vi "Generator DC Sweep Manager.vi"(8 "error in (no error)":errorcluster, 10 "sweep index":i32=-1, 11 "Lockin.DAQ in":refnum<class "Lockin.DAQ.lvclass">) -> (0 "error out":errorcluster, 2 "Array":waveform(dbl)[](array[waveform]), 3 "Lockin.DAQ out":refnum<class "Lockin.DAQ.lvclass">)   [LabVIEW 2019, in "Lockin.DAQ.lvclass"]
uses:
  Lockin.DAQ.lvclass
  Lockin.DAQ.lvclass/Lockin.DAQ.ctl
panel:
  out "time":dbl
  out "sweeping":dbl
  out "start sweep time":timestamp
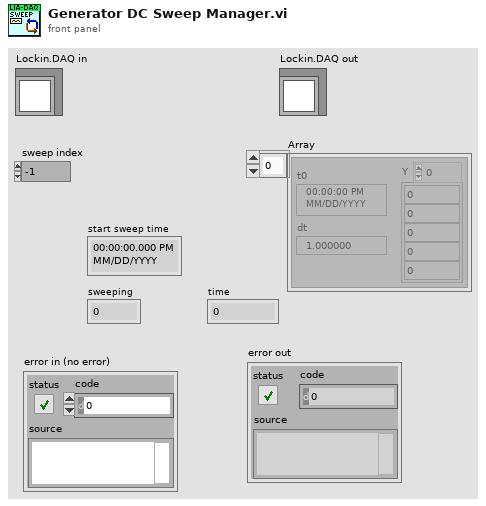
[diagram p1: front panel]
types:
  T1 = typedef "Lockin.DAQ.lvclass/Sampling.ctl" = cluster{"Fs":dbl, "#s":i32}
  T2 = typedef "Lockin.DAQ.lvclass/AO-cluster.ctl" = T3[]
  T3 = typedef "Instrument.Lockin.UI.lvclass/AO Channel--Cluster.ctl" = cluster{"Enable?":bool, "Channel":i32, "Amplitude":dbl, "Offset":dbl, "Frequency":dbl, "Phase":dbl, "Function":T4, "Sweeping?":bool}
  T4 = typedef "Lockin.DAQ.lvclass/Function-enum.ctl" = enum16{"Sine", "Triangle", "Square"}
  T5 = typedef "Instrument.Lockin.UI.lvclass/Sweep Channel--Cluster.ctl" = cluster{"End":dbl, "Start":dbl, "Channel":u16, "Pattern":T6}
  T6 = typedef "Lockin.DAQ.lvclass/Sweep Pattern--Enum.ctl" = enum16{"Ramp /", "Ramp /\\", "Smooth Ramp _/", "Smooth Ramp _/\\_", "Frequency"}
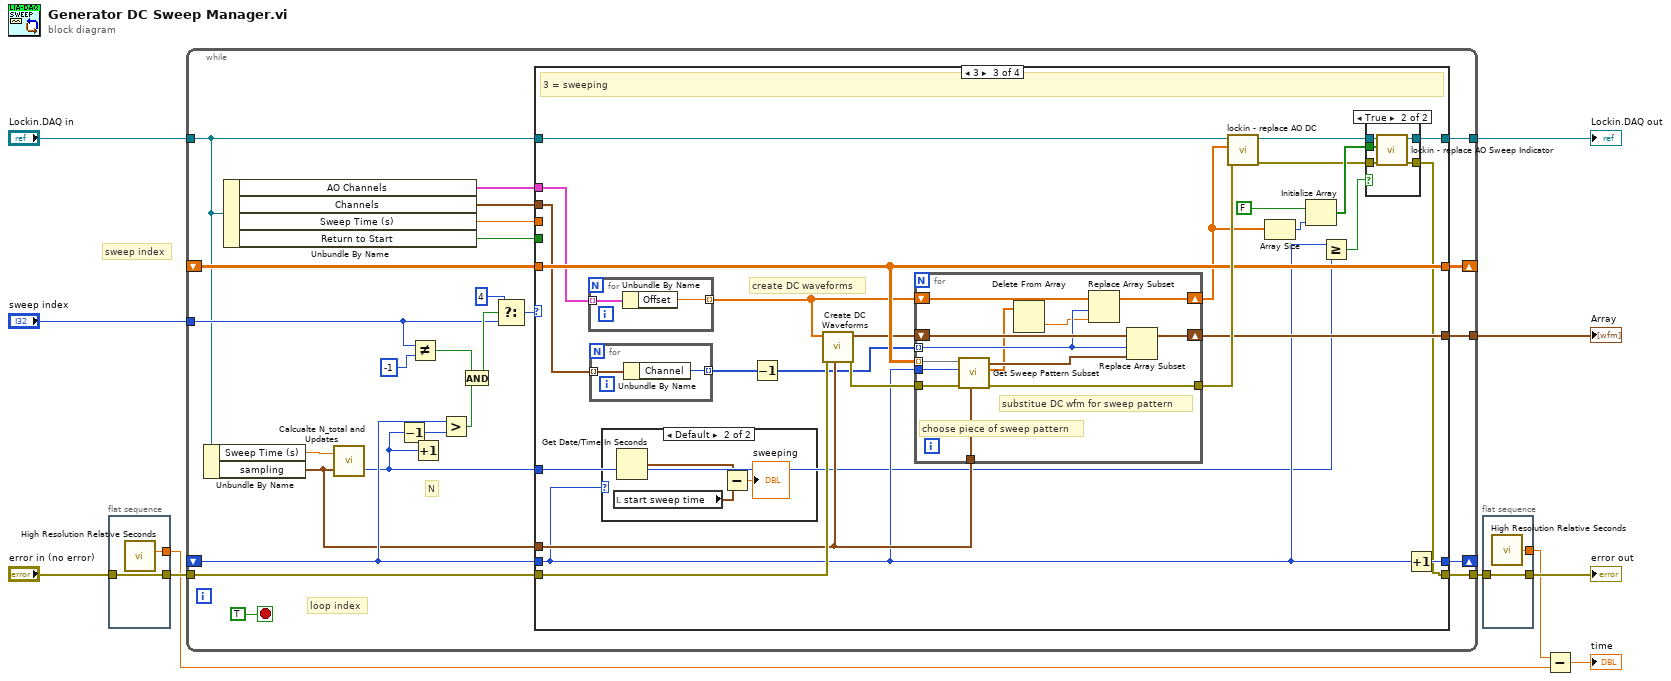
[diagram p0: block diagram]
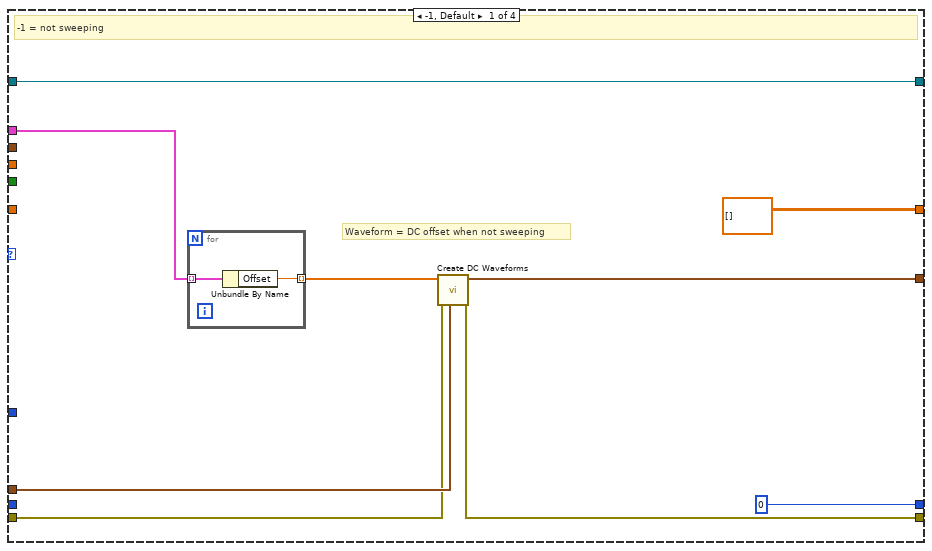
[diagram p2: hidden frame]
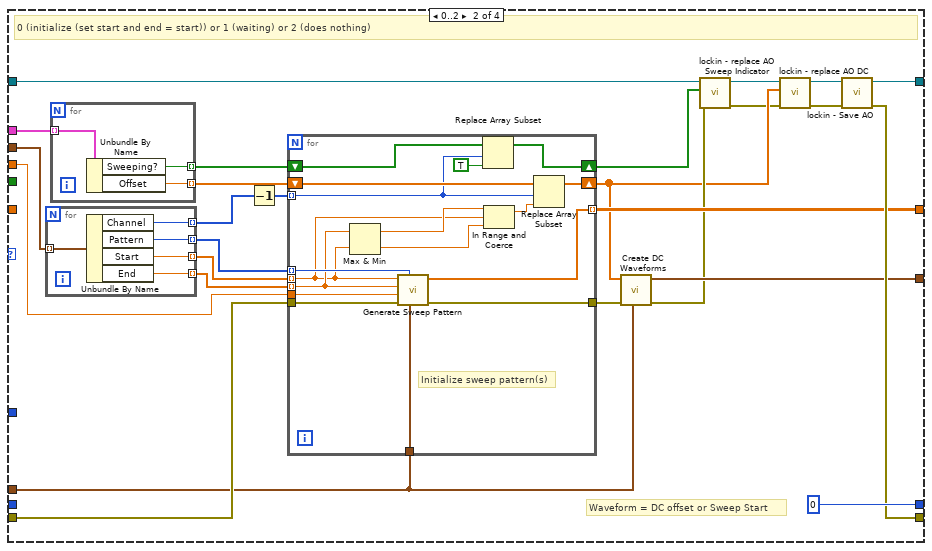
[diagram p3: hidden frame]
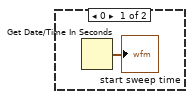
[diagram p5: hidden frame]
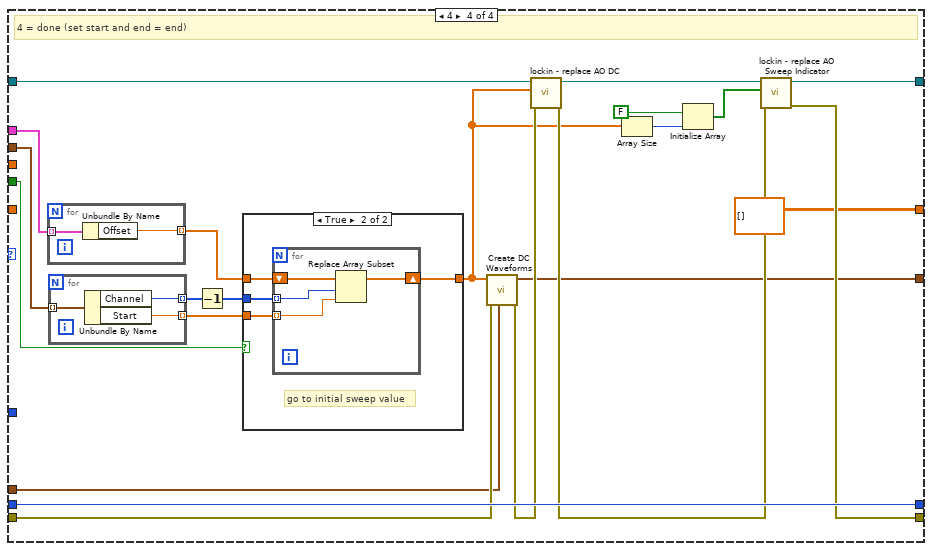
[diagram p6: hidden frame]
diagram:
  # "sweep index"
  n1 = flat-sequence {
    tunnel: "error in (no error)" -> [w13]
    tunnel: [w13] -> w7
    tunnel: [w12] -> w4
    frame #0 {
      n2 = call <vilib>:"High Resolution Relative Seconds.vi"() -> ("relative seconds"=w12:dbl)
    }
  }
  n3 = while {
    tunnel: "sweep index" -> [w21]
    shift-right: [w38] -> _
    shift-left: _ -> [w32]
    tunnel: [w35] -> w10
    tunnel: "Lockin.DAQ in" -> [w18]
    tunnel: w7 -> [w34]
    tunnel: [w33] -> w5
    shift-right: [w29] -> _
    shift-left: _ -> [w27]
    tunnel: [w30] -> w2
    stop <- TRUE stop-if-true
    # "N"
    # "loop index"
    n4 = Unbundle By Name(w18) -> ("Sweep Time (s)"=w26:dbl, "sampling"=w25:T1)
    n5 = Unbundle By Name(w18) -> ("AO Channels"=w17:T2, "Channels"=w16:T5[], "Sweep Time (s)"=w15:dbl, "Return to Start"=w14:bool)
    n6 = call "Calcualte N_total and Updates.vi"("Sampling"=w25, "Sweep Time (s)"=w26) -> ("Updates"=w20:i32)  [unwired: 1 out]
    n7 = Decrement(x=w20) -> (x-1=w19:i32)
    n8 = Not Equal?(x=w21, y=-1 ("x")) -> (x != y?=w23:bool)
    n9 = Increment(x=w20) -> ()  [unwired: 1 out]
    n10 = Greater?(x=w32, y=w19) -> (0:w31:bool)
    n11 = And(x=w23, y=w31) -> (x .and. y?=w24:bool)
    n12 = Select(t=4, s=w24, f=w21) -> (s? t:f=w36:i32)
    n13 = case shown="3" w36 {
      tunnel: [0 0 w125 w173] -> w38
      tunnel: w32 -> [_ _ w105 w173]
      tunnel: w20 -> [_ _ w104 _]
      tunnel: [w41 w73 w111 w172] -> w35
      tunnel: w34 -> [w44 w69 w121 w168]
      tunnel: [w43 w72 w107 w171] -> w33
      tunnel: w25 -> [w45 w66 w119 w166]
      tunnel: [w42 w67 w116 w165] -> w30
      tunnel: [dbl[][] [] ("Sweep Pattern") w70 w123 dbl[][] [] ("Sweep Pattern")] -> w29
      tunnel: w27 -> [_ _ w123 _]
      tunnel: w18 -> [w41 w57 w115 w159]
      tunnel: w17 -> [w39 w56 w103 w155]
      tunnel: w16 -> [_ w55 w101 w157]
      tunnel: w15 -> [_ w54 _ _]
      tunnel: w14 -> [_ _ _ w156]
      frame -1, Default {
        # "Waveform = DC offset when not sweeping"
        # "-1 = not sweeping"
        n14 = for {
          tunnel: w39 -> [w49] mode=indexing
          tunnel: [w48] -> w40 mode=indexing
          n15 = Unbundle By Name(w49) -> ("Offset"=w48:dbl)
        }
        n16 = call "Create DC Waveforms.vi"("sampling"=w45, "error in (no error)"=w44, "DC (V)"=w40) -> ("Error out"=w43:errorcluster, "Waveforms []"=w42:waveform(dbl)[])  [unwired: 7 in]
      }
      frame 0..2 {
        # "Waveform = DC offset or Sweep Start"
        # "0 (initialize (set start and end = start)) or 1 (waiting) or 2 (does nothing)"
        n17 = for {
          tunnel: [w80] -> w53 mode=indexing
          tunnel: [w79] -> w52 mode=indexing
          tunnel: [w78] -> w51 mode=indexing
          tunnel: [w77] -> w50 mode=indexing
          tunnel: w55 -> [w76] mode=indexing
          n18 = Unbundle By Name(w76) -> ("Channel"=w77:u16, "Pattern"=w78:T6, "Start"=w79:dbl, "End"=w80:dbl)
        }
        n19 = for {
          tunnel: [w83] -> w68 mode=indexing
          tunnel: [w82] -> w63 mode=indexing
          tunnel: w56 -> [w81] mode=indexing
          n20 = Unbundle By Name(w81) -> ("Sweeping?"=w82:bool, "Offset"=w83:dbl)
        }
        n21 = Decrement(x=w50) -> (x-1=w75:u16[])
        n22 = for {
          shift-right: [w99] -> w62
          shift-left: w68 -> [w100]
          tunnel: w53 -> [w85] mode=indexing
          tunnel: w52 -> [w84] mode=indexing
          tunnel: w75 -> [w92] mode=indexing
          shift-right: [w97] -> w71
          shift-left: w63 -> [w87]
          tunnel: w54 -> [w96]
          tunnel: w69 -> [w95]
          tunnel: w66 -> [w94]
          tunnel: [w93] -> w70 mode=indexing
          tunnel: [w88] -> w65
          tunnel: w51 -> [w86] mode=indexing
          # "Initialize sweep pattern(s)"
          n23 = Max & Min(x=w85, y=w84) -> (max(x,y)=w91:dbl, min(x,y)=w90:dbl)
          n24 = call "Generate Sweep Pattern.vi"("Sampling"=w94, "Sweep Pattern"=w86, "error in (no error)"=w95, "Sweep Lockin Time (s)"=w96, "Sweep End"=w85, "Sweep Start"=w84) -> ("error out"=w88:errorcluster, "Sweep Pattern"=w93:dbl[])  [unwired: 4 in]
          n25 = Replace Array Subset(array=w87, new element=TRUE ("new element/subarray"), index=w92) -> (w97:bool[])
          n26 = In Range and Coerce(upper limit=w91, x=w84, lower limit=w90) -> (coerced(x)=w98:dbl)  [unwired: 1 out]
          n27 = Replace Array Subset(array=w100, new element=w98, index=w92) -> (w99:dbl[])
        }
        n28 = call "Create DC Waveforms.vi"("sampling"=w66, "error in (no error)"=w65, "DC (V)"=w62) -> ("Error out"=w64:errorcluster, "Waveforms []"=w67:waveform(dbl)[])  [unwired: 7 in]
        n29 = call "lockin - replace AO Sweep Indicator.vi"("error in (no error)"=w64, "Channels: AO.Sweep?"=w71, "Lockin.DAQ"=w57) -> ("error out"=w59:errorcluster, "Lockin.DAQ out"=w60:refnum<class "Lockin.DAQ.lvclass">)  [unwired: 7 in]
        n30 = call "lockin - replace AO DC.vi"("error in (no error)"=w59, "AO.DC (V)"=w62, "Lockin.DAQ"=w60) -> ("error out"=w58:errorcluster, "Lockin.DAQ out"=w61:refnum<class "Lockin.DAQ.lvclass">)  [unwired: 7 in]
        n31 = call "lockin - Save AO.vi"("error in (no error)"=w58, "Lockin.DAQ"=w61) -> ("error out"=w72:errorcluster, "Lockin.DAQ out"=w73:refnum<class "Lockin.DAQ.lvclass">)  [unwired: 8 in]
      }
      frame 3 {
        # "create DC waveforms"
        # "3 = sweeping"
        n32 = for {
          tunnel: [w129] -> w117 mode=indexing
          tunnel: w103 -> [w128] mode=indexing
          n33 = Unbundle By Name(w128) -> ("Offset"=w129:dbl)
        }
        n34 = for {
          tunnel: [w127] -> w102 mode=indexing
          tunnel: w101 -> [w126] mode=indexing
          n35 = Unbundle By Name(w126) -> ("Channel"=w127:u16)
        }
        n36 = case shown="Default" w105 {
          frame 0 {
            n37 = Get Date/Time In Seconds() -> (seconds since 1Jan1904=→"start sweep time":timestamp)
          }
          frame Default {
            n38 = local read "start sweep time"() -> (w152:timestamp)
            n39 = Get Date/Time In Seconds() -> (seconds since 1Jan1904=w151:timestamp)
            n40 = Subtract(x=w151, y=w152) -> (x-y=→"sweeping":dbl)
          }
        }
        n41 = Decrement(x=w102) -> (x-1=w118:u16[])
        n42 = call "Create DC Waveforms.vi"("sampling"=w119, "error in (no error)"=w121, "DC (V)"=w117) -> ("Error out"=w120:errorcluster, "Waveforms []"=w122:waveform(dbl)[])  [unwired: 7 in]
        n43 = for {
          tunnel: w119 -> [w145]
          tunnel: w123 -> [w149] mode=indexing
          tunnel: w105 -> [w148]
          tunnel: w120 -> [w147]
          tunnel: [w146] -> w124
          shift-right: [w142] -> w116
          shift-left: w122 -> [w144]
          tunnel: w118 -> [w140] mode=indexing
          shift-right: [w139] -> w109
          shift-left: w117 -> [w141]
          # "substitue DC wfm for sweep pattern"
          # "choose piece of sweep pattern"
          n44 = call "Get Sweep Pattern Subset.vi"("Sampling"=w145, "error in (no error)"=w147, "index"=w148, "Sweep Pattern"=w149) -> ("error out"=w146:errorcluster, "Pattern Subset"=w138:dbl[], "output waveform"=w143:waveform(dbl))  [unwired: 5 in]
          n45 = Delete From Array(array=w138) -> (deleted portion=w137:dbl)  [unwired: 2 in, 1 out]
          n46 = Replace Array Subset(array=w141, new element=w137, index=w140) -> (w139:dbl[])
          n47 = Replace Array Subset(array=w144, new element=w143, index=w140) -> (w142:waveform(dbl)[])
        }
        n48 = call "lockin - replace AO DC.vi"("error in (no error)"=w124, "AO.DC (V)"=w109, "Lockin.DAQ"=w115) -> ("error out"=w108:errorcluster, "Lockin.DAQ out"=w112:refnum<class "Lockin.DAQ.lvclass">)  [unwired: 7 in]
        n49 = Array Size(array=w109) -> (size(s)=w110:i32)
        n50 = Initialize Array(FALSE, w110) -> (w113:bool[])
        n51 = Greater Or Equal?(x=w105, y=w104) -> (x >= y?=w106:bool)
        n52 = case shown="True" w106 {
          tunnel: w113 -> [_ w136]
          tunnel: w112 -> [w131 w135]
          tunnel: [w131 w134] -> w111
          tunnel: w108 -> [w130 w133]
          tunnel: [w130 w132] -> w107
          frame False {
          }
          frame True {
            n53 = call "lockin - replace AO Sweep Indicator.vi"("error in (no error)"=w133, "Channels: AO.Sweep?"=w136, "Lockin.DAQ"=w135) -> ("error out"=w132:errorcluster, "Lockin.DAQ out"=w134:refnum<class "Lockin.DAQ.lvclass">)  [unwired: 7 in]
          }
        }
        n54 = Increment(x=w105) -> (x+1=w125:i32)
      }
      frame 4 {
        # "4 = done (set start and end = end)"
        n55 = for {
          tunnel: [w177] -> w154 mode=indexing
          tunnel: w155 -> [w176] mode=indexing
          n56 = Unbundle By Name(w176) -> ("Offset"=w177:dbl)
        }
        n57 = for {
          tunnel: [w180] -> w175 mode=indexing
          tunnel: [w179] -> w160 mode=indexing
          tunnel: w157 -> [w178] mode=indexing
          n58 = Unbundle By Name(w178) -> ("Channel"=w179:u16, "Start"=w180:dbl)
        }
        n59 = Decrement(x=w160) -> (x-1=w174:u16[])
        n60 = case shown="True" w156 {
          tunnel: w175 -> [_ w185]
          tunnel: w174 -> [_ w184]
          tunnel: w154 -> [w181 w183]
          tunnel: [w181 w182] -> w161
          frame False {
            # "remain at current value of DC"
          }
          frame True {
            # "go to initial sweep value"
            n61 = for {
              shift-right: [w186] -> w182
              shift-left: w183 -> [w189]
              tunnel: w185 -> [w188] mode=indexing
              tunnel: w184 -> [w187] mode=indexing
              n62 = Replace Array Subset(array=w189, new element=w188, index=w187) -> (w186:dbl[])
            }
          }
        }
        n63 = call "Create DC Waveforms.vi"("sampling"=w166, "error in (no error)"=w168, "DC (V)"=w161) -> ("Error out"=w167:errorcluster, "Waveforms []"=w165:waveform(dbl)[])  [unwired: 7 in]
        n64 = call "lockin - replace AO DC.vi"("error in (no error)"=w167, "AO.DC (V)"=w161, "Lockin.DAQ"=w159) -> ("error out"=w169:errorcluster, "Lockin.DAQ out"=w170:refnum<class "Lockin.DAQ.lvclass">)  [unwired: 7 in]
        n65 = Array Size(array=w161) -> (size(s)=w163:i32)
        n66 = Initialize Array(FALSE, w163) -> (w162:bool[])
        n67 = call "lockin - replace AO Sweep Indicator.vi"("error in (no error)"=w169, "Channels: AO.Sweep?"=w162, "Lockin.DAQ"=w170) -> ("error out"=w171:errorcluster, "Lockin.DAQ out"=w172:refnum<class "Lockin.DAQ.lvclass">)  [unwired: 7 in]
      }
    }
  }
  "Lockin.DAQ out" <- w10
  "Array" <- w2
  n68 = flat-sequence {
    tunnel: w5 -> [w191]
    tunnel: [w191] -> w6
    tunnel: [w190] -> w1
    frame #0 {
      n69 = call <vilib>:"High Resolution Relative Seconds.vi"() -> ("relative seconds"=w190:dbl)
    }
  }
  n70 = Subtract(x=w1, y=w4) -> (x-y=→"time":dbl)
  "error out" <- w6
